vi "AIT 1553 - Filter Acyclic Frames.vi"(8 "error in (no error)":errorcluster, 10 "Bus Controller Page Item Refs in":T1[](array[typedef]) format="%.0x") -> (0 "error out":errorcluster, 2 "Bus Controller Page Message Section Refs out":T1[](array[typedef]) format="%.0x", 3 "Bus Controller Page Acyclic Frame Refs out":T1[](array[typedef]) format="%.0x")   [LabVIEW 2011, in "AIT 1553 Custom Device.lvlib"]
uses:
  <vilib>/NI Veristand/Custom Device API/Custom Device Item Ref.ctl
  AIT 1553 Custom Device.lvlib
  <vilib>/NI Veristand/Custom Device API/Custom Device API.lvlib
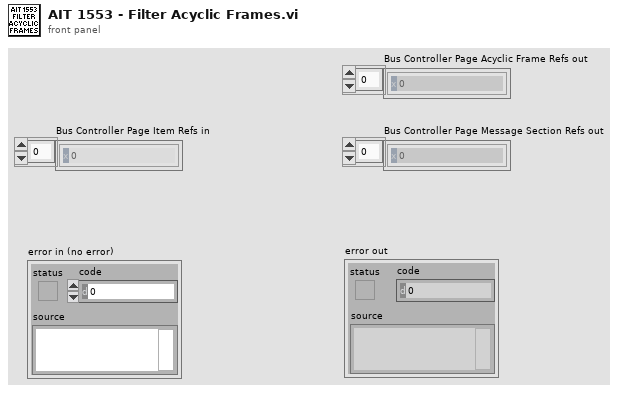
[diagram p1: front panel]
types:
  T1 = typedef "Custom Device API.lvlib/Custom Device Item Ref.ctl" = u64
  T2 = typedef "Custom Device API.lvlib/Custom Device Item Info.ctl" = cluster{"Name":string, "Is Channel":bool, "GUID":string}
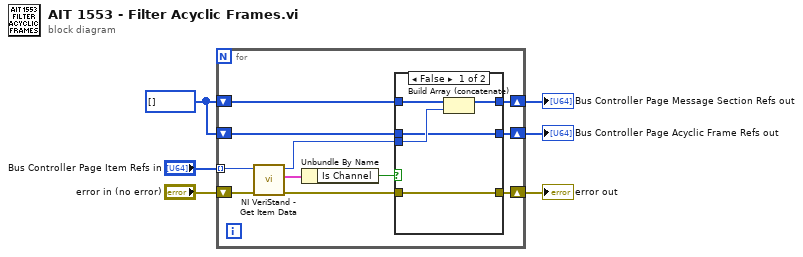
[diagram p0: block diagram]
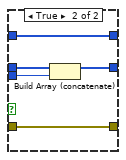
[diagram p2: hidden frame]
diagram:
  w3 = T1[] [] ("Bus Controller Page Item Refs in")
  n1 = for {
    shift-right: [w14] -> w4
    shift-left: "error in (no error)" -> [w16]
    tunnel: "Bus Controller Page Item Refs in" -> [w17] mode=indexing
    shift-right: [w9] -> w2
    shift-left: w3 -> [w11]
    shift-right: [w7] -> w1
    shift-left: w3 -> [w10]
    n2 = call <vilib>:"NI VeriStand - Get Item Data.vi"("error in (no error)"=w16, "Item Ref in"=w17) -> ("error out"=w15:errorcluster, "Item Info"=w13:T2, "Item Ref out"=w8:T1)  [unwired: 6 in, 1 out]
    n3 = Unbundle By Name(w13) -> ("Is Channel"=w12:bool)
    n4 = case shown="False" w12 {
      tunnel: [w18 w27] -> w14
      tunnel: w15 -> [w18 w27]
      tunnel: w11 -> [w22 w26]
      tunnel: w10 -> [w19 w25]
      tunnel: [w20 w26] -> w9
      tunnel: w8 -> [w21 w24]
      tunnel: [w19 w23] -> w7
      frame False {
        n5 = Build Array (concatenate)(w22, w21) -> (w20:T1[])
      }
      frame True {
        n6 = Build Array (concatenate)(w25, w24) -> (w23:T1[])
      }
    }
  }
  "Bus Controller Page Message Section Refs out" <- w2
  "Bus Controller Page Acyclic Frame Refs out" <- w1
  "error out" <- w4
